vi "斯坦道XML解析.vi"(9 "工作状态":u16, 10 "添加的路径":path, 11 "参数簇":cluster{"id":u16, "flowid":dbl, "range":dbl}={"id"=1, "flowid"=0.0, "range"=0.0}) -> (1 "简易步骤名称":string, 2 "步骤时间":string[](array[string]), 3 "步骤名":string[](array[string]))   [LabVIEW 2016, in "斯坦道CODcr.lvlib"]
uses:
  <vilib>/xml/Load XML File.vi
  <vilib>/xml/Close Reference(Node).vi
  <resource>/objmgr/DOMUserDefRef.rc
  <vilib>/xml/NI_XML.lvlib
panel:
  out "连接的字符串":string
  out "大小":i32
  out "XML字符串":string="<?xml version=\"1.0\" encoding=\"ISO-8859-1\"?>\n<bookstore>\n<book ISBN=\"978-0545128285\">\n  <title lang=\"en\">The Tales of Beedle the Bard</title>\n  <author>J. K. Rowling</author>\n  <year>2008</year>\n  <price>12.99</price>\n</book>\n<book ISBN=\"978-0316160209\">\n  <title lang=\"en\">Eclipse</title>\n  <author>Stephenie Meyer</author>\n  <year>2007</year>\n  <price>19.99</price>\n</book>\n<book ISBN=\"978-0316067928\">\n  <title lang=\"en\">Breaking Dawn</title>\n  <author>Stephenie Meyer</author>\n  <year>2008</year>\n  <price>22.99</price>\n</book>\n<book ISBN=\"978-0316017923\">\n  <title lang=\"en\">Outliers: The Story of Success</title>\n  <author>Malcolm Gladwell</author>\n  <year>2008</year>\n  <price>27.99</price>\n</book>\n<book ISBN=\"978-0596007645\">\n  <title lang=\"en\">XML in a Nutshell</title>\n  <author>Elliotte Rusty Harold</author>\n  <author>W. Scott Means</author>\n  <year>2004</year>\n  <price>39.95</price>\n</book>\n</bookstore>"
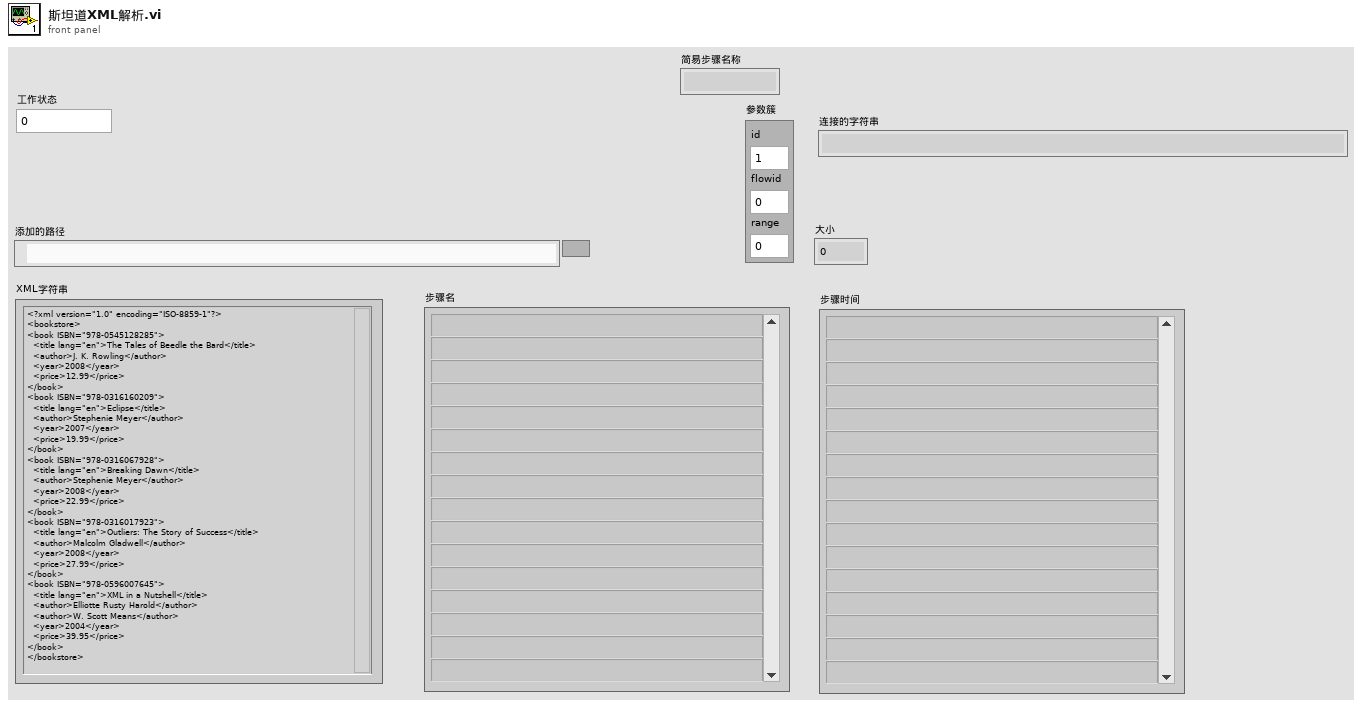
[diagram p1: front panel]
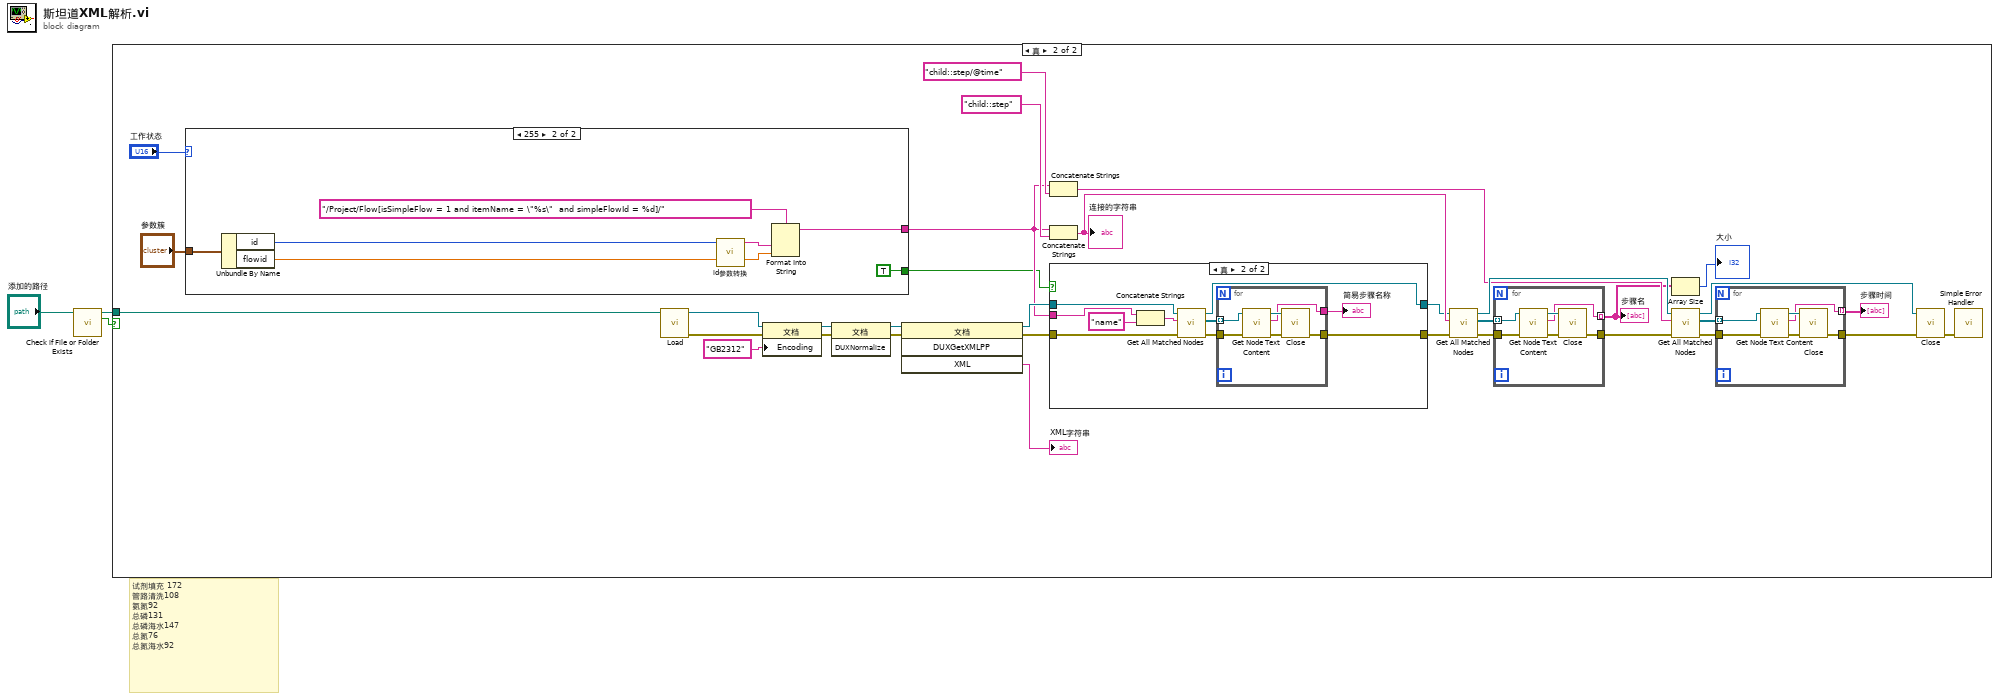
[diagram p0: block diagram]
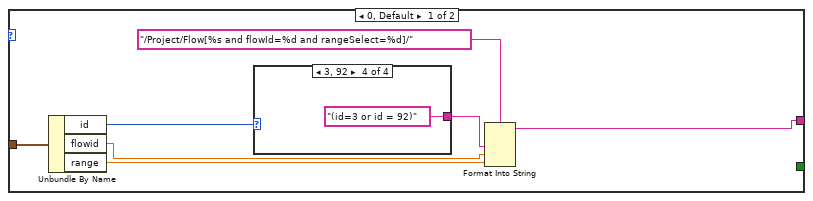
[diagram p4: hidden frame]
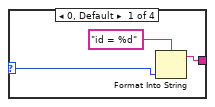
[diagram p5: hidden frame]
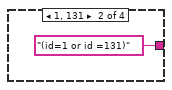
[diagram p6: hidden frame]
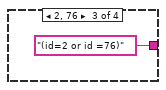
[diagram p7: hidden frame]
diagram:
  # "试剂填充 172 \n管路清洗108\n氨氮92\n总磷131\n总磷海水147\n总氮76\n总氮海水92"
  n1 = call <vilib>:"Check if File or Folder Exists.vi"("path"="添加的路径") -> ("file or folder exists?"=w1:bool, "dup path"=w2:path)  [unwired: 8 in, 1 out]
  n2 = case shown="真" w1 {
    tunnel: w2 -> [_ w24]
    frame False {
    }
    frame True {
      n3 = case shown="255" "工作状态" {
        tunnel: "参数簇" -> [w61 w74]
        tunnel: [w57 w71] -> w6
        tunnel: [_ TRUE] -> w4
        frame 0, Default {
          n4 = Unbundle By Name(w61) -> ("id"=w56:u16, "flowid"=w59:dbl, "range"=w58:dbl)
          n5 = case shown="3, 92" w56 {
            selector: w56 -> [w63 _ _ _]
            tunnel: [w62 "(id=1 or id =131)" ("输入 4") "(id=2 or id =76)" ("输入 4") "(id=3 or id = 92)" ("输入 4")] -> w55
            frame 0, Default {
              n6 = Format Into String(format string="id = %d" ("格式字符串"), w63) -> (resulting string=w62:string)  [unwired: 2 in, 1 out]
            }
            frame 1, 131 {
            }
            frame 2, 76 {
            }
            frame 3, 92 {
            }
          }
          n7 = Format Into String(format string="/Project/Flow[%s and flowId=%d and rangeSelect=%d]/" ("XPath expression"), w55, w59, w58) -> (resulting string=w57:string)  [unwired: 2 in, 1 out]
        }
        frame 255 {
          n8 = Unbundle By Name(w74) -> ("id"=w70:u16, "flowid"=w72:dbl)
          n9 = call "id参数转换.vi"("id"=w70) -> ("table输出"=w69:string)  [unwired: 9 in, 1 out]
          n10 = Format Into String(format string="/Project/Flow[isSimpleFlow = 1 and itemName = \"%s\"  and simpleFlowId = %d]/" ("XPath expression"), w69, w72) -> (resulting string=w71:string)  [unwired: 2 in, 1 out]
        }
      }
      n11 = call-poly <vilib>:"Load.vi"("path to XML document"=w24) -> ("DOM document out"=w32:refnum<k20>, "error out"=w31:errorcluster)  [unwired: 12 in, 1 out]
      n12 = property on="属性节点" class="文档"(reference=w32, error in=w31, "Encoding"="GB2312" ("文档编码")) -> (reference out=w30:refnum<k20>, error out=w29:errorcluster)
      n13 = invoke on="Invoke Node" class="文档" method="DUXNormalize"(reference=w30, error in=w29) -> (reference out=w27:refnum<k20>, error out=w28:errorcluster)  [unwired: 1 in, 1 out]
      n14 = invoke on="Invoke Node" class="文档" method="DUXGetXMLPP"(reference=w27, error in=w28) -> (reference out=w9:refnum<k20>, error out=w8:errorcluster, "XML"=→"XML字符串":string)  [unwired: 2 in, 1 out]
      n15 = Concatenate Strings(w6, "child::step/@time" ("输入 4")) -> (w13:string)
      n16 = Concatenate Strings(w6, "child::step" ("输入 4")) -> (w15:string)
      "连接的字符串" <- w15
      n17 = case shown="真" w4 {
        tunnel: w9 -> [w38 w48]
        tunnel: w8 -> [w37 w47]
        tunnel: [w38 w46] -> w7
        tunnel: w6 -> [_ w44]
        tunnel: [w37 w40] -> w5
        frame False {
        }
        frame True {
          n18 = Concatenate Strings(w44, "name" ("输入 4")) -> (w43:string)
          n19 = call <vilib>:"Get All Matched Nodes.vi"("error in (no error)"=w47, "XPath expression"=w43, "node in"=w48) -> ("error out"=w41:errorcluster, "node result array"=w42:refnum<k20>[], "node out"=w46:refnum<k20>)  [unwired: 6 in]
          n20 = for {
            tunnel: w41 -> [w54]
            tunnel: [w51] -> w39
            tunnel: w42 -> [w50] mode=indexing
            tunnel: [w49] -> w40
            n21 = call <vilib>:"Get Node Text Content.vi"("error in (no error)"=w54, "node in"=w50) -> ("error out"=w52:errorcluster, "node text"=w51:string, "node out"=w53:refnum<k20>)  [unwired: 7 in]
            n22 = call-poly <vilib>:"Close.vi"("error in (no error)"=w52, "node"=w53) -> ("error out"=w49:errorcluster)  [unwired: 7 out]
          }
          "简易步骤名称" <- w39
        }
      }
      n23 = call <vilib>:"Get All Matched Nodes.vi"("error in (no error)"=w5, "XPath expression"=w15, "node in"=w7) -> ("error out"=w23:errorcluster, "node result array"=w22:refnum<k20>[], "node out"=w19:refnum<k20>)  [unwired: 6 in]
      n24 = for {
        tunnel: w23 -> [w86]
        tunnel: [w83] -> w12 mode=indexing
        tunnel: w22 -> [w82] mode=indexing
        tunnel: [w81] -> w18
        n25 = call <vilib>:"Get Node Text Content.vi"("error in (no error)"=w86, "node in"=w82) -> ("error out"=w84:errorcluster, "node text"=w83:string, "node out"=w85:refnum<k20>)  [unwired: 7 in]
        n26 = call-poly <vilib>:"Close.vi"("error in (no error)"=w84, "node"=w85) -> ("error out"=w81:errorcluster)  [unwired: 7 out]
      }
      "步骤名" <- w12
      n27 = Array Size(array=w12) -> (size(s)=→"大小":i32)
      n28 = call <vilib>:"Get All Matched Nodes.vi"("error in (no error)"=w18, "XPath expression"=w13, "node in"=w19) -> ("error out"=w21:errorcluster, "node result array"=w20:refnum<k20>[], "node out"=w25:refnum<k20>)  [unwired: 6 in]
      n29 = for {
        tunnel: w21 -> [w80]
        tunnel: [w77] -> w17 mode=indexing
        tunnel: w20 -> [w76] mode=indexing
        tunnel: [w75] -> w26
        n30 = call <vilib>:"Get Node Text Content.vi"("error in (no error)"=w80, "node in"=w76) -> ("error out"=w78:errorcluster, "node text"=w77:string, "node out"=w79:refnum<k20>)  [unwired: 7 in]
        n31 = call-poly <vilib>:"Close.vi"("error in (no error)"=w78, "node"=w79) -> ("error out"=w75:errorcluster)  [unwired: 7 out]
      }
      "步骤时间" <- w17
      n32 = call-poly <vilib>:"Close.vi"("error in (no error)"=w26, "node"=w25) -> ("error out"=w36:errorcluster)  [unwired: 7 out]
      n33 = call <vilib>:"Simple Error Handler.vi"("error in (no error)"=w36) -> ()  [unwired: 4 in, 5 out]
    }
  }
